vi "Finish.vi"   [LabVIEW 2019]
doc: "This VI is called just before exiting. It is expected to close I/O refnum, save collected data, etc."
types:
  T1 = typedef "WPI_JoystickDevRef.ctl" = cluster{"Device":T2}
  T2 = typedef "WPI_JoystickDeviceEnum.ctl" = enum16{"USB 0", "USB 1", "USB 2", "USB 3", "USB 4", "USB 5"}
  T3 = typedef "WPI_RobotDriveDevRef.ctl" = cluster{"DevStatus":errorcluster, "Motors[]":T4[], "Square Inputs":bool, "Max Output":dbl}
  T4 = typedef "WPI_MotorControlDeviceRef.ctl" = cluster{"DeviceStatus":errorcluster, "Type":T5, "PWM":cluster{"PWM Channel":T6, "DeadBand":T7}, "CAN":cluster{"Device Number":u8, "SetOutput VI Ref":variant, "GetOutput VI Ref":variant, "Enable VI Ref":variant, "Disable VI Ref":variant, "Data":variant}, "Invert":bool, "DIO PWM":cluster{"PWM \"Enable\" Channel":T6, "DIOChannel":T8, "PWM Rate":dbl}}
  T5 = typedef "WPI_MotorControlType.ctl" = enum16{"PWM", "CAN", "DIO PWM"}
  T6 = typedef "FPGA_DIOPWMChannel.ctl" = enum8{"PWM 0", "PWM 1", "PWM 2", "PWM 3", "PWM 4", "PWM 5", "PWM 6", "PWM 7", "PWM 8", "PWM 9", "PWM MXP 0", "PWM MXP 1", "PWM MXP 2", "PWM MXP 3", "PWM MXP 4", "PWM MXP 5", "PWM MXP 6", "PWM MXP 7", "PWM MXP 8", "PWM MXP 9", "Invalid"}
  T7 = typedef "WPI_PWMDeadband.ctl" = cluster{"Name":string, "maxPositivePwm":i32, "minPositivePwm":i32, "centerPwm":i32, "maxNegativePwm":i32, "minNegativePwm":i32, "angularRange":u16}
  T8 = typedef "FPGA_DIOChannel.ctl" = enum8{"DIO 0", "DIO 1", "DIO 2", "DIO 3", "DIO 4", "DIO 5", "DIO 6", "DIO 7", "DIO 8", "DIO 9", "DIO MXP 0", "DIO MXP 1", "DIO MXP 2", "DIO MXP 3", "DIO MXP 4", "DIO MXP 5", "DIO MXP 6", "DIO MXP 7", "DIO MXP 8", "DIO MXP 9", "DIO MXP 10", "DIO MXP 11", "DIO MXP 12", "DIO MXP 13", "DIO MXP 14", "DIO MXP 15", "SPI Port CS1", "SPI Port CS2", "SPI Port CS3", "SPI Port MISO", "SPI Port MOSI", "Invalid"}
  T9 = typedef "WPI_PotentiometerDevRef.ctl" = cluster{"DevStatus":errorcluster, "Analog Channel":T10, "Invert Output":bool}
  T10 = typedef "FPGA_AIChannel.ctl" = enum8{"AI 0", "AI 1", "AI 2", "AI 3", "AI MXP 0", "AI MXP 1", "AI MXP 2", "AI MXP 3", "Invalid"}
  T11 = typedef "WPI_ServoDeviceRef.ctl" = cluster{"DeviceStatus":errorcluster, "PWM Channel":T6, "DeadBand":T7}
  T12 = typedef "WPI_SwitchDevRef.ctl" = cluster{"DevStatus":errorcluster, "DIO Channel":T8, "CntIndex":T13, "Normally Closed":bool}
  T13 = typedef "FPGA_CounterCtrSystemIndex.ctl" = enum8{"Ctr 0", "Ctr 1", "Ctr 2", "Ctr 3", "Ctr 4", "Ctr 5", "Ctr 6", "Ctr 7", "Invalid"}
  T14 = typedef "WPI_AccelerometerDevRef.ctl" = cluster{"DevStatus":errorcluster, "Scaling":T15, "Analog Channels":T16, "I2C Bus":T17, "SPI Bus":T18, "Accel Range":T19, "ADXL Axes":T20, "Handle":i32, "Device Address":u8, "Accel Type":enum16{"Analog", "ADXL345 I2C", "ADXL345 SPI", "Internal", "ADXL362 SPI"}}
  T15 = typedef "WPI_AccelerometerScaling.ctl" = cluster{"Gain (VoltsPerG)":dbl, "Center Voltage":dbl}
  T16 = typedef "WPI_AccelerometerAnalogChannels.ctl" = cluster{"X-Axis":T10, "Y-Axis":T10, "Z-Axis":T10}
  T17 = typedef "i2c_bus.ctl" = enum16{"I2C On-Board", "I2C MXP", "Invalid"}
  T18 = typedef "spi_bus.ctl" = enum16{"SPI On-Board, CS0", "SPI On-Board, CS1", "SPI On-Board, CS2", "SPI On-Board, CS3", "SPI MXP", "Invalid"}
  T19 = typedef "ADXL345 Range.ctl" = u8
  T20 = typedef "WPI_AccelerometerADXL345 Axes.ctl" = cluster{"X-Axis":bool, "Y-Axis":bool, "Z-Axis":bool}
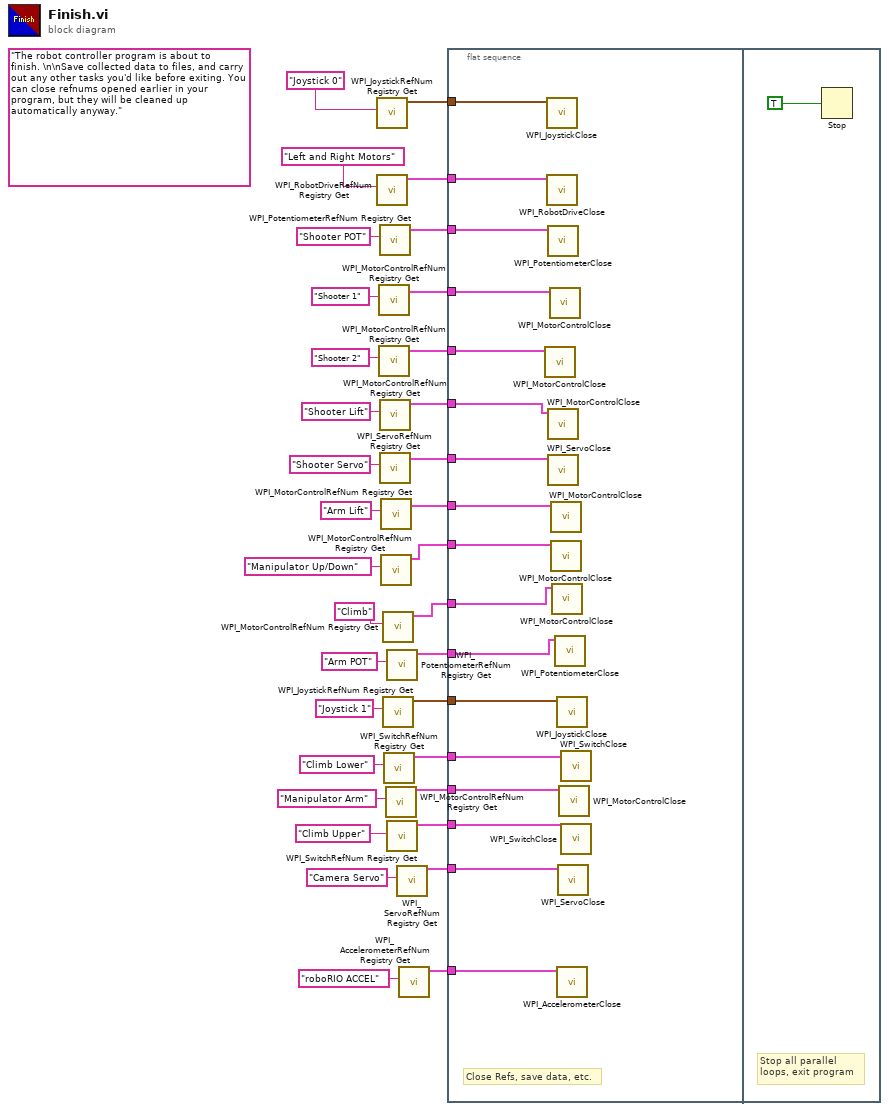
[diagram p0: block diagram]
diagram:
  (unwired) "The robot controller program is about to finish. \n\nSave collected data to files, and carry out any other tasks you'd like before exiting. You can close refnums opened earlier in your program, but they will be cleaned up automatically anyway."
  n1 = call <vilib>:"WPI_JoystickRefNum Registry Get.vi"("refnum name"="Joystick 0") -> ("JoystickDevRef"=w31:T1)  [unwired: 1 in, 9 out]
  n2 = call <vilib>:"WPI_RobotDriveRefNum Registry Get.vi"("refnum name"="Left and Right Motors") -> ("RobotDriveDevRef"=w32:T3)  [unwired: 1 in, 9 out]
  n3 = call <vilib>:"WPI_MotorControlRefNum Registry Get.vi"("refnum name"="Shooter 1") -> ("MotorControlDevRef"=w28:T4)  [unwired: 9 in, 1 out]
  n4 = call <vilib>:"WPI_MotorControlRefNum Registry Get.vi"("refnum name"="Shooter 2") -> ("MotorControlDevRef"=w26:T4)  [unwired: 9 in, 1 out]
  n5 = call <vilib>:"WPI_PotentiometerRefNum Registry Get.vi"("refnum name"="Shooter POT") -> ("PotDevRef"=w30:T9)  [unwired: 9 in, 1 out]
  n6 = call <vilib>:"WPI_MotorControlRefNum Registry Get.vi"("refnum name"="Shooter Lift") -> ("MotorControlDevRef"=w24:T4)  [unwired: 9 in, 1 out]
  n7 = call <vilib>:"WPI_ServoRefNum Registry Get.vi"("refnum name"="Shooter Servo") -> ("ServoDeviceRef"=w22:T11)  [unwired: 9 in, 1 out]
  n8 = call <vilib>:"WPI_MotorControlRefNum Registry Get.vi"("refnum name"="Arm Lift") -> ("MotorControlDevRef"=w18:T4)  [unwired: 9 in, 1 out]
  n9 = call <vilib>:"WPI_MotorControlRefNum Registry Get.vi"("refnum name"="Manipulator Up/Down") -> ("MotorControlDevRef"=w19:T4)  [unwired: 9 in, 1 out]
  n10 = call <vilib>:"WPI_MotorControlRefNum Registry Get.vi"("refnum name"="Climb") -> ("MotorControlDevRef"=w20:T4)  [unwired: 9 in, 1 out]
  n11 = call <vilib>:"WPI_JoystickRefNum Registry Get.vi"("refnum name"="Joystick 1") -> ("JoystickDevRef"=w12:T1)  [unwired: 9 in, 1 out]
  n12 = call <vilib>:"WPI_SwitchRefNum Registry Get.vi"("refnum name"="Climb Lower") -> ("SwitchDevRef"=w9:T12)  [unwired: 9 in, 1 out]
  n13 = call <vilib>:"WPI_MotorControlRefNum Registry Get.vi"("refnum name"="Manipulator Arm") -> ("MotorControlDevRef"=w6:T4)  [unwired: 9 in, 1 out]
  n14 = call <vilib>:"WPI_PotentiometerRefNum Registry Get.vi"("refnum name"="Arm POT") -> ("PotDevRef"=w14:T9)  [unwired: 9 in, 1 out]
  n15 = call <vilib>:"WPI_SwitchRefNum Registry Get.vi"("refnum name"="Climb Upper") -> ("SwitchDevRef"=w10:T12)  [unwired: 9 in, 1 out]
  n16 = call <vilib>:"WPI_ServoRefNum Registry Get.vi"("refnum name"="Camera Servo") -> ("ServoDeviceRef"=w4:T11)  [unwired: 9 in, 1 out]
  n17 = call <vilib>:"WPI_AccelerometerRefNum Registry Get.vi"("refnum name"="roboRIO ACCEL") -> ("AccelerometerDevRef"=w1:T14)  [unwired: 9 in, 1 out]
  n18 = flat-sequence {
    tunnel: w32 -> [w51]
    tunnel: w31 -> [w50]
    tunnel: w30 -> [w49]
    tunnel: w28 -> [w48]
    tunnel: w26 -> [w47]
    tunnel: w24 -> [w46]
    tunnel: w22 -> [w45]
    tunnel: w20 -> [w44]
    tunnel: w19 -> [w43]
    tunnel: w18 -> [w42]
    tunnel: w14 -> [w41]
    tunnel: w12 -> [w40]
    tunnel: w10 -> [w39]
    tunnel: w9 -> [w38]
    tunnel: w6 -> [w37]
    tunnel: w4 -> [w36]
    tunnel: w1 -> [w35]
    frame #0 {
      # "Close Refs, save data, etc."
      n19 = call <vilib>:"WPI_MotorControlClose.vi"("MotorControlDevRef"=w47) -> ()  [unwired: 10 in, 1 out]
      n20 = call <vilib>:"WPI_JoystickClose.vi"("JoystickDevRef"=w50) -> ()  [unwired: 11 out]
      n21 = call <vilib>:"WPI_RobotDriveClose.vi"("RobotDriveDevRef"=w51) -> ()  [unwired: 1 in, 10 out]
      n22 = call <vilib>:"WPI_PotentiometerClose.vi"("PotDevRef"=w49) -> ()  [unwired: 10 in, 1 out]
      n23 = call <vilib>:"WPI_MotorControlClose.vi"("MotorControlDevRef"=w46) -> ()  [unwired: 10 in, 1 out]
      n24 = call <vilib>:"WPI_ServoClose.vi"("ServoDeviceRef"=w45) -> ()  [unwired: 10 in, 1 out]
      n25 = call <vilib>:"WPI_MotorControlClose.vi"("MotorControlDevRef"=w48) -> ()  [unwired: 10 in, 1 out]
      n26 = call <vilib>:"WPI_MotorControlClose.vi"("MotorControlDevRef"=w42) -> ()  [unwired: 10 in, 1 out]
      n27 = call <vilib>:"WPI_MotorControlClose.vi"("MotorControlDevRef"=w43) -> ()  [unwired: 10 in, 1 out]
      n28 = call <vilib>:"WPI_MotorControlClose.vi"("MotorControlDevRef"=w44) -> ()  [unwired: 10 in, 1 out]
      n29 = call <vilib>:"WPI_PotentiometerClose.vi"("PotDevRef"=w41) -> ()  [unwired: 10 in, 1 out]
      n30 = call <vilib>:"WPI_JoystickClose.vi"("JoystickDevRef"=w40) -> ()  [unwired: 11 in]
      n31 = call <vilib>:"WPI_AccelerometerClose.vi"("AccelerometerDevRef"=w35) -> ()  [unwired: 10 in, 1 out]
      n32 = call <vilib>:"WPI_ServoClose.vi"("ServoDeviceRef"=w36) -> ()  [unwired: 10 in, 1 out]
      n33 = call <vilib>:"WPI_MotorControlClose.vi"("MotorControlDevRef"=w37) -> ()  [unwired: 10 in, 1 out]
      n34 = call <vilib>:"WPI_SwitchClose.vi"("SwitchDevRef"=w38) -> ()  [unwired: 10 in, 1 out]
      n35 = call <vilib>:"WPI_SwitchClose.vi"("SwitchDevRef"=w39) -> ()  [unwired: 10 in, 1 out]
    }
    frame #1 {
      # "Stop all parallel\nloops, exit program"
      n36 = Stop(stop? (T)=TRUE ("Quit")) -> ()
    }
  }
